vi "Query RF Connection Information.vi"(8 "error in (no error)":errorcluster, 10 "RF Connection (\"RF1.1\")":string="RF1.1", 11 "VISA resource name":refnum<visa-resource-name>) -> (0 "error out":errorcluster, 2 "Information":string, 3 "VISA resource name out":refnum<visa-resource-name>)   [LabVIEW 2015, in "Rohde&Schwarz CMXP Base.lvlib"]
doc: "Returns information about the specified signal path.\n\nAttribute:\n-\n\nRemote-control command:\n[CONFigure:]TENVironment:SPATh:INFO?"
uses:
  <instrlib>/Rohde&Schwarz CMXP Base/Rohde&Schwarz CMXP Base.lvlib
  <instrlib>/Rohde&Schwarz CMXP Base/Private/rsidr_core.llb/rsidr_core.lvlib
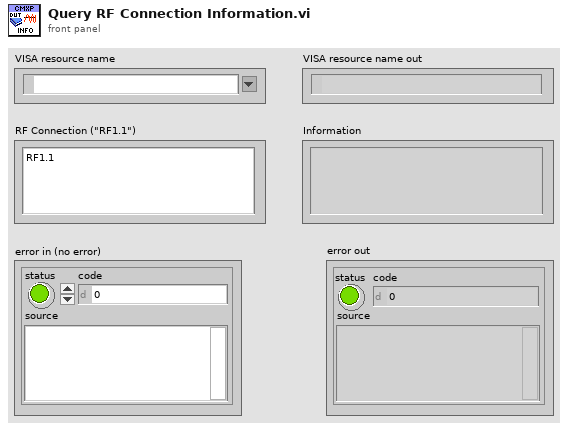
[diagram p1: front panel]
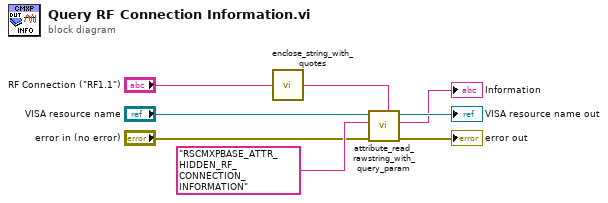
[diagram p0: block diagram]
diagram:
  n1 = call <instrlib>:"enclose_string_with_quotes.vi"("String to enclose"="RF Connection (\"RF1.1\")") -> ("String out"=w1:string)  [unwired: 4 in]
  n2 = call <instrlib>:"attribute_read_rawstring_with_query_param.vi"("Query Parameter (None)"=w1, "error in"="error in (no error)", "Attribute ID"="RSCMXPBASE_ATTR_HIDDEN_RF_CONNECTION_INFORMATION", "VISA resource name"="VISA resource name") -> ("error out"=→"error out":errorcluster, "RawString out"=→"Information":string, "VISA resource name out"=→"VISA resource name out":refnum<visa-resource-name>)  [unwired: 5 in]
